vi "Get Temperature.vi"(4 "Channel":i32, 8 "error in (no error)":errorcluster, 11 "Instrument.Oxford1820 in":refnum<class "Instrument.Oxford1820.lvclass">) -> (0 "error out":errorcluster, 1 "Status":variant, 2 "Temperature (K)":dbl, 3 "Instrument.Oxford1820 out":refnum<class "Instrument.Oxford1820.lvclass">)   [LabVIEW 2016, in "Instrument.Oxford1820.lvclass"]
uses:
  Instrument.Oxford1820.lvclass
  <userlib>/LevyLab/Levylab Instruments/Instrument Types/Cryostat/Instrument.Cryostat.lvclass
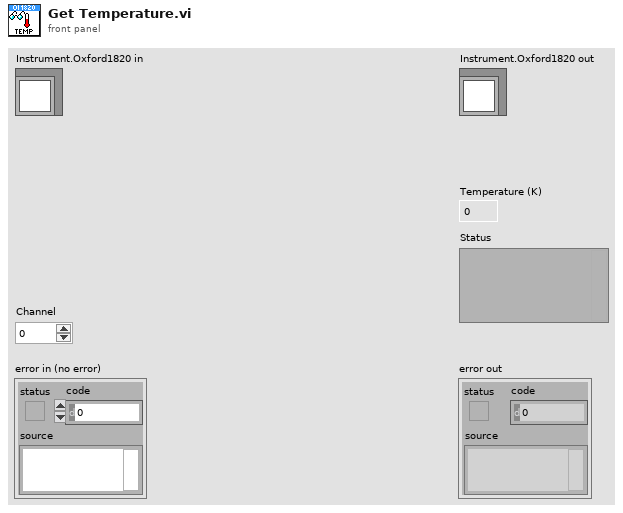
[diagram p1: front panel]
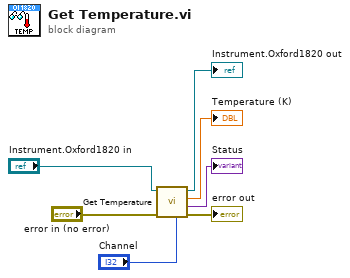
[diagram p0: block diagram]
diagram:
  n1 = call-parent "Get Temperature.vi"("Channel"="Channel", "error in (no error)"="error in (no error)", "Instrument.Cryostat in"="Instrument.Oxford1820 in") -> ("error out"=→"error out":errorcluster, "Status"=→"Status":variant, "Temperature (K)"=→"Temperature (K)":dbl, "Instrument.Cryostat out"=→"Instrument.Oxford1820 out":refnum<class "Instrument.Oxford1820.lvclass">)  [unwired: 5 in]
